vi "Swerve Wheel.vi"(2 "Wheel":T1(ring), 4 "Inputs":dbl[](array[numeric])) -> (0 "Speed":dbl)   [LabVIEW 2018]
uses:
  <vilib>/Rock Robotics/Network Tables/NT Read Number.vi
  <vilib>/addons/control/pid/pid.llb/PID (DBL).vi
  <vilib>/Rock Robotics/Network Tables/NT Write Number.vi
  <vilib>/addons/control/pid/NI_PID_pid.lvlib
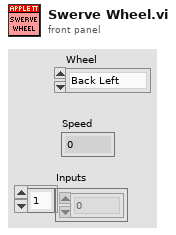
[diagram p1: front panel]
types:
  T1 = enum16{"Back Left", "Back Right", "Front Left", "Front Right"}
  T2 = enum16{"Z", "Y", "X", "Rot. Point X", "Rot. Point Y", "Width/2", "Max", "Length/2"}
  T3 = enum16{"Z Axis", "Y", "X", "Rot. Point X", "Rot. Point Y", "Width/2", "Max", "Length/2"}
  T4 = cluster{"proportional gain (Kc)":dbl, "integral time (Ti, min)":dbl, "derivative time (Td, min)":dbl}
  T5 = typedef "WPI_AnalogChannelDevRef.ctl" = cluster{"DevStatus":errorcluster, "Analog Channel":T6}
  T6 = typedef "FPGA_AIChannel.ctl" = enum8{"AI 0", "AI 1", "AI 2", "AI 3", "AI MXP 0", "AI MXP 1", "AI MXP 2", "AI MXP 3", "Invalid"}
  T7 = typedef "WPI_MotorControlDeviceRef.ctl" = cluster{"DeviceStatus":errorcluster, "Type":T8, "PWM":cluster{"PWM Channel":T9, "DeadBand":T10}, "CAN":cluster{"Device Number":u8, "SetOutput VI Ref":variant, "GetOutput VI Ref":variant, "Enable VI Ref":variant, "Disable VI Ref":variant, "Data":variant}, "Invert":bool, "DIO PWM":cluster{"PWM \"Enable\" Channel":T9, "DIOChannel":T11, "PWM Rate":dbl}}
  T8 = typedef "WPI_MotorControlType.ctl" = enum16{"PWM", "CAN", "DIO PWM"}
  T9 = typedef "FPGA_DIOPWMChannel.ctl" = enum8{"PWM 0", "PWM 1", "PWM 2", "PWM 3", "PWM 4", "PWM 5", "PWM 6", "PWM 7", "PWM 8", "PWM 9", "PWM MXP 0", "PWM MXP 1", "PWM MXP 2", "PWM MXP 3", "PWM MXP 4", "PWM MXP 5", "PWM MXP 6", "PWM MXP 7", "PWM MXP 8", "PWM MXP 9", "Invalid"}
  T10 = typedef "WPI_PWMDeadband.ctl" = cluster{"Name":string, "maxPositivePwm":i32, "minPositivePwm":i32, "centerPwm":i32, "maxNegativePwm":i32, "minNegativePwm":i32, "angularRange":u16}
  T11 = typedef "FPGA_DIOChannel.ctl" = enum8{"DIO 0", "DIO 1", "DIO 2", "DIO 3", "DIO 4", "DIO 5", "DIO 6", "DIO 7", "DIO 8", "DIO 9", "DIO MXP 0", "DIO MXP 1", "DIO MXP 2", "DIO MXP 3", "DIO MXP 4", "DIO MXP 5", "DIO MXP 6", "DIO MXP 7", "DIO MXP 8", "DIO MXP 9", "DIO MXP 10", "DIO MXP 11", "DIO MXP 12", "DIO MXP 13", "DIO MXP 14", "DIO MXP 15", "SPI Port CS1", "SPI Port CS2", "SPI Port CS3", "SPI Port MISO", "SPI Port MOSI", "Invalid"}
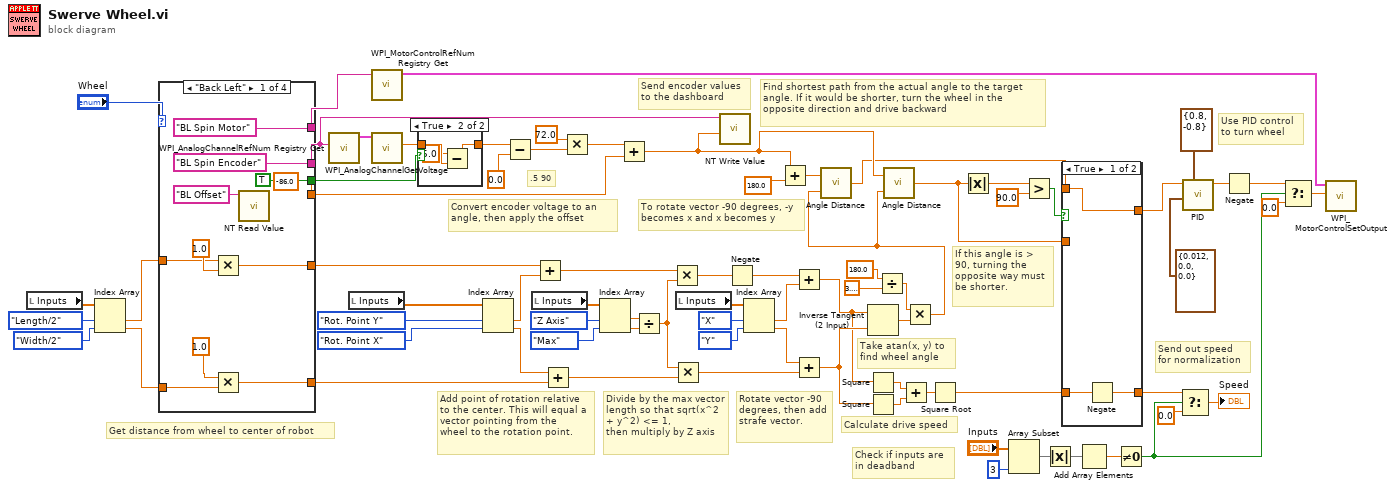
[diagram p0: block diagram]
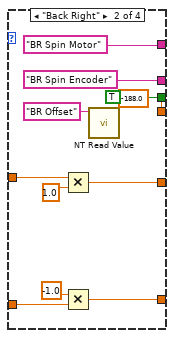
[diagram p4: hidden frame]
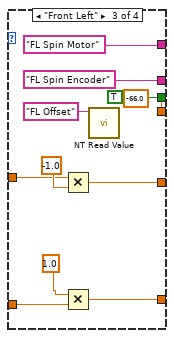
[diagram p5: hidden frame]
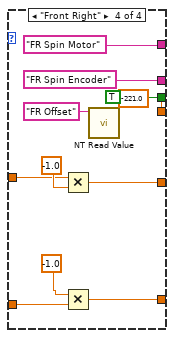
[diagram p6: hidden frame]
diagram:
  # ".5 90"
  # "Send encoder values \nto the dashboard"
  # "To rotate vector -90 degrees, -y becomes x and x becomes y"
  # "Divide by the max vector length so that sqrt(x^2 + y^2) <= 1,\nthen multiply by Z axis"
  # "Add point of rotation relative to the center. This will equal a vector pointing from the\nwheel to the rotation point."
  # "Send out speed\nfor normalization"
  # "Check if inputs are\nin deadband"
  # "Convert encoder voltage to an angle, then apply the offset"
  # "If this angle is > 90, turning the opposite way must be shorter."
  # "Use PID control\nto turn wheel"
  # "Find shortest path from the actual angle to the target angle. If it would be shorter, turn the wheel in the opposite direction and drive backward"
  # "Take atan(x, y) to find wheel angle"
  # "Calculate drive speed"
  # "Rotate vector -90 degrees, then add strafe vector."
  # "Get distance from wheel to center of robot"
  n1 = local read "Inputs"() -> (w14:dbl[])
  n2 = Index Array(array=w14, index #1=T2."Length/2", index #2=T2."Width/2") -> (element #1=w12:dbl, element #2=w11:dbl)
  n3 = case shown="\"Back Left\"" "Wheel" {
    tunnel: ["BL Spin Encoder" "BR Spin Encoder" "FL Spin Encoder" "FR Spin Encoder"] -> w41
    tunnel: ["BL Spin Motor" "BR Spin Motor" "FL Spin Motor" "FR Spin Motor"] -> w61
    tunnel: [-86.0 ("Numeric") -188.0 ("Numeric") -66.0 ("Numeric") -221.0 ("Numeric")] -> w52
    tunnel: w12 -> [w83 w94 w105 w116]
    tunnel: w11 -> [w81 w92 w103 w114]
    tunnel: [w80 w91 w102 w113] -> w38
    tunnel: [w79 w90 w101 w112] -> w34
    tunnel: [TRUE TRUE TRUE TRUE] -> w1
    frame "Back Left" {
      n4 = Multiply(x=w83, y=1.0) -> (x*y=w80:dbl)
      n5 = Multiply(x=1.0 ("y"), y=w81) -> (x*y=w79:dbl)
      n6 = call-poly <vilib>:"NT Read Value.vi"("Name"="BL Offset") -> ()  [unwired: 9 in, 2 out]
    }
    frame "Back Right" {
      n7 = Multiply(x=w94, y=1.0) -> (x*y=w91:dbl)
      n8 = Multiply(x=-1.0 ("y"), y=w92) -> (x*y=w90:dbl)
      n9 = call-poly <vilib>:"NT Read Value.vi"("Name"="BR Offset") -> ()  [unwired: 9 in, 2 out]
    }
    frame "Front Left" {
      n10 = Multiply(x=w105, y=-1.0) -> (x*y=w102:dbl)
      n11 = Multiply(x=1.0 ("y"), y=w103) -> (x*y=w101:dbl)
      n12 = call-poly <vilib>:"NT Read Value.vi"("Name"="FL Offset") -> ()  [unwired: 9 in, 2 out]
    }
    frame "Front Right" {
      n13 = Multiply(x=w116, y=-1.0) -> (x*y=w113:dbl)
      n14 = Multiply(x=-1.0 ("y"), y=w114) -> (x*y=w112:dbl)
      n15 = call-poly <vilib>:"NT Read Value.vi"("Name"="FR Offset") -> ()  [unwired: 9 in, 2 out]
    }
  }
  n16 = call <vilib>:"WPI_AnalogChannelRefNum Registry Get.vi"("refnum name"=w41) -> ("AIDeviceRef"=w56:T5)  [unwired: 9 in, 1 out]
  n17 = local read "Inputs"() -> (w36:dbl[])
  n18 = call <vilib>:"WPI_MotorControlRefNum Registry Get.vi"("refnum name"=w61) -> ("MotorControlDevRef"=w74:T7)  [unwired: 9 in, 1 out]
  n19 = call <vilib>:"WPI_AnalogChannelGetVoltage.vi"("AIDeviceRef"=w56) -> ("Voltage"=w2:dbl)  [unwired: 8 in, 2 out]
  n20 = case shown="True" w1 {
    tunnel: [w121 w124] -> w3
    tunnel: w2 -> [w121 w123]
    frame False {
    }
    frame True {
      n21 = Subtract(x=5.0, y=w123) -> (x-y=w124:dbl)
    }
  }
  n22 = Index Array(array=w36, index #1=T2."Rot. Point Y", index #2=T2."Rot. Point X") -> (element #1=w32:dbl, element #2=w33:dbl)
  n23 = Subtract(x=w3, y=0.0) -> (x-y=w55:dbl)
  n24 = local read "Inputs"() -> (w30:dbl[])
  n25 = Add(x=w38, y=w32) -> (x+y=w7:dbl)
  n26 = Add(x=w33, y=w34) -> (x+y=w26:dbl)
  n27 = Multiply(x=72.0 ("y"), y=w55) -> (x*y=w53:dbl)
  n28 = Index Array(array=w30, index #1=T3."Z Axis", index #2=T2."Max") -> (element #1=w27:dbl, element #2=w28:dbl)
  n29 = Add(x=w53, y=w52) -> (x+y=w5:dbl)
  n30 = Divide(x=w27, y=w28) -> (x/y=w25:dbl)
  n31 = Multiply(x=w7, y=w25) -> (x*y=w9:dbl)
  n32 = Multiply(x=w25, y=w26) -> (x*y=w20:dbl)
  n33 = local read "Inputs"() -> (w23:dbl[])
  n34 = call-poly <vilib>:"NT Write Value.vi"("Numeric"=w5, "Name"=w41) -> ()  [unwired: 9 in, 1 out]
  n35 = Negate(x=w9) -> (-x=w8:dbl)
  n36 = Index Array(array=w23, index #1=T2."X", index #2=T2."Y") -> (element #1=w18:dbl, element #2=w19:dbl)
  n37 = Add(x=w5, y=180.0 ("f")) -> (x+y=w48:dbl)
  n38 = Add(x=w8, y=w18) -> (x+y=w16:dbl)
  n39 = Add(x=w19, y=w20) -> (x+y=w17:dbl)
  n40 = Inverse Tangent (2 Input)(1:w17, 2:w16) -> (0:w72:dbl)
  n41 = Square(x=w16) -> (x^2=w21:dbl)
  n42 = Square(x=w17) -> (x^2=w71:dbl)
  n43 = Divide(x=180.0 ("y"), y=3.141592653589793) -> (x/y=w69:dbl)
  n44 = Add(x=w21, y=w71) -> (x+y=w70:dbl)
  n45 = Multiply(x=w69, y=w72) -> (x*y=w10:dbl)
  n46 = call "Angle Distance.vi"("target angle"=w10, "current angle"=w48) -> ("distance"=w4:dbl)
  n47 = call "Angle Distance.vi"("target angle"=w10, "current angle"=w5) -> ("distance"=w63:dbl)
  n48 = Square Root(x=w70) -> (sqrt(x)=w62:dbl)
  n49 = Absolute Value(x=w63) -> (abs(x)=w64:dbl)
  n50 = Array Subset(array="Inputs", length=3) -> (w47:dbl[])  [unwired: 1 in]
  n51 = Greater?(x=w64, y=90.0) -> (0:w43:bool)
  n52 = Absolute Value(x=w47) -> (abs(x)=w39:dbl[])
  n53 = case shown="True" w43 {
    tunnel: w4 -> [w125 _]
    tunnel: w63 -> [_ w129]
    tunnel: [w126 w128] -> w46
    tunnel: w62 -> [w127 w128]
    tunnel: [w125 w129] -> w58
    frame True {
      n54 = Negate(x=w127) -> (-x=w126:dbl)
    }
    frame False {
    }
  }
  n55 = Add Array Elements(numeric array=w39) -> (sum=w73:dbl)
  n56 = Not Equal To 0?(x=w73) -> (x != 0?=w42:bool)
  n57 = Select(t=w46, s=w42, f=0.0) -> (s? t:f=→"Speed":dbl)
  n58 = call-poly <vilib>:"PID.vi"("output range"=cluster{"output high":dbl, "output low":dbl} {"output high"=0.8, "output low"=-0.8}, "PID gains"=T4 {"proportional gain (Kc)"=0.012, "integral time (Ti, min)"=0.0, "derivative time (Td, min)"=0.0}, "setpoint"=w58) -> ("output"=w50:dbl)  [unwired: 7 in, 1 out]
  n59 = Negate(x=w50) -> (-x=w40:dbl)
  n60 = Select(t=w40, s=w42, f=0.0) -> (s? t:f=w51:dbl)
  n61 = call <vilib>:"WPI_MotorControlSetOutput.vi"("Output"=w51, "MotorControlDevRef"=w74) -> ()  [unwired: 7 in, 3 out]
